vi "Recursively List All Files.vi"(9 "File Key Word":string, 11 "Folder Path":path) -> (3 "Files":path[](array[path]))   [LabVIEW 2024]
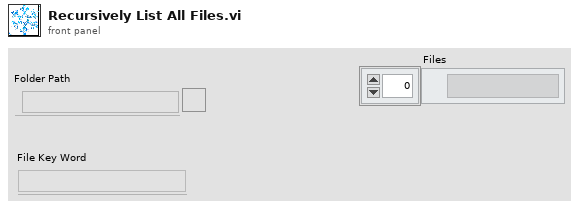
[diagram p1: front panel]
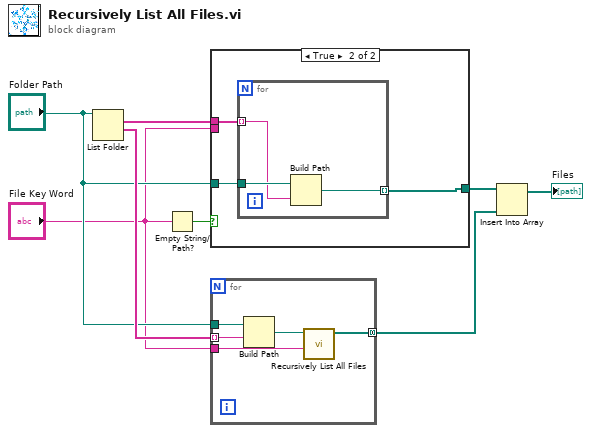
[diagram p0: block diagram]
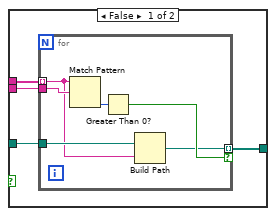
[diagram p2: hidden frame]
diagram:
  n1 = List Folder(path="Folder Path") -> (filenames=w8:string[], folder names=w6:string[])  [unwired: 3 in, 2 out]
  n2 = Empty String/Path?(string/path="File Key Word") -> (empty?=w7:bool)
  n3 = case shown="True" w7 {
    tunnel: w8 -> [w12 w21]
    tunnel: "File Key Word" -> [w11 _]
    tunnel: [w9 w19] -> w3
    tunnel: "Folder Path" -> [w10 w20]
    frame False {
      n4 = for {
        tunnel: w12 -> [w14] mode=indexing
        tunnel: w11 -> [w17]
        tunnel: [w13] -> w9 mode=indexing if=w18
        tunnel: w10 -> [w15]
        n5 = Match Pattern(string=w14, regular expression=w17) -> (offset past match=w16:i32)  [unwired: 1 in, 3 out]
        n6 = Greater Than 0?(x=w16) -> (x > 0?=w18:bool)
        n7 = Build Path(base path=w15, name or relative path=w14) -> (appended path=w13:path)
      }
    }
    frame True {
      n8 = for {
        tunnel: w21 -> [w23] mode=indexing
        tunnel: w20 -> [w24]
        tunnel: [w22] -> w19 mode=indexing
        n9 = Build Path(base path=w24, name or relative path=w23) -> (appended path=w22:path)
      }
    }
  }
  n10 = for {
    tunnel: w6 -> [w29] mode=indexing
    tunnel: "Folder Path" -> [w28]
    tunnel: "File Key Word" -> [w26]
    tunnel: [w25] -> w1 mode=concatenating
    n11 = Build Path(base path=w28, name or relative path=w29) -> (appended path=w27:path)
    n12 = call "Recursively List All Files.vi"("File Key Word"=w26, "Folder Path"=w27) -> ("Files"=w25:path[])  [unwired: 9 in]
  }
  n13 = Insert Into Array(array=w3, new element=w1) -> (→"Files":path[])  [unwired: 1 in]
